vi "Map IO.vi"(8 "error in":errorcluster, 9 "Input":u8[](array[numeric]), 10 "Output":u8[](array[numeric]), 11 "SL_SC in":refnum<class "SL_SC.lvclass">) -> (0 "error out":errorcluster, 1 "Boolean Array":bool[](array[boolean]), 2 "Port Array":u8[](array[numeric]), 3 "SL_SC out":refnum<class "SL_SC.lvclass">)   [LabVIEW 2019, in "SL_SC.lvlib" / "SL_SC.lvclass"]
uses:
  Library/SL_SC.lvclass
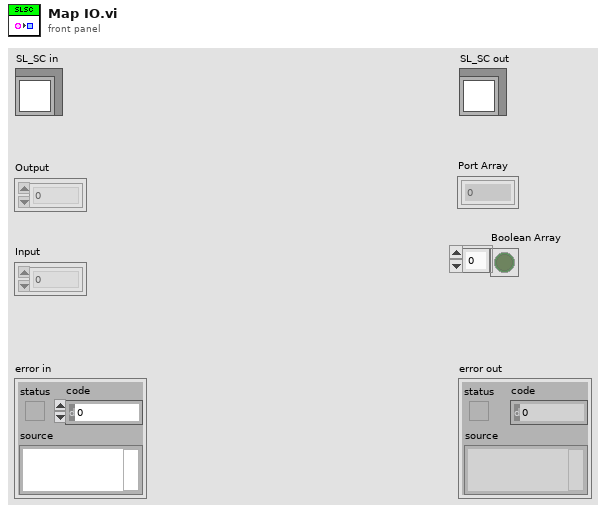
[diagram p1: front panel]
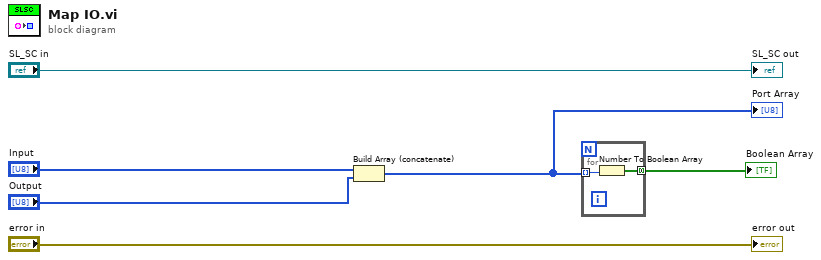
[diagram p0: block diagram]
diagram:
  n1 = Build Array (concatenate)("Input", "Output") -> (w1:u8[])
  "Port Array" <- w1
  n2 = for {
    tunnel: w1 -> [w8] mode=indexing
    tunnel: [w7] -> w4 mode=concatenating
    n3 = Number To Boolean Array(number=w8) -> (Boolean array=w7:bool[])
  }
  "Boolean Array" <- w4
  "error out" <- "error in"
  "SL_SC out" <- "SL_SC in"
